vi "SP_ZAction.vi"(8 "error in (no error)":errorcluster, 10 "Z Action":T1(ring), 11 "SemiProbe in":refnum<class "SemiProbe.lvclass">) -> (0 "error out":errorcluster, 1 "previous Z [µm]":i32, 2 "Z [µm]":i32, 3 "SemiProbe out":refnum<class "SemiProbe.lvclass">)   [LabVIEW 2019, in "SemiProbe.lvclass"]
uses:
  SemiProbe.lvclass
  InstrumentSetup.vi
  <vilib>/Utility/error.llb/Error Cluster From Error Code.vi
  <vilib>/ErrorRing/Error Ring.xnode
  ArduinoControl/ArduinoControl.lvclass
  InstrControl.lvclass
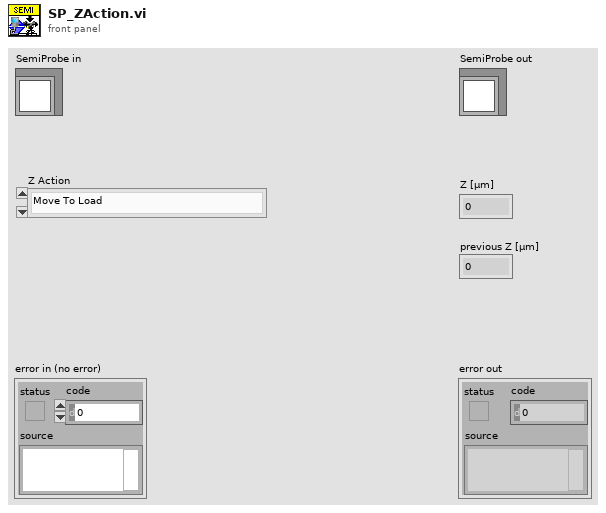
[diagram p1: front panel]
types:
  T1 = enum16{"Move To Load", "Move To Double Separation", "Move To Separation Distance", "Move To Contact", "Execute Contact Search", "Execute Arduino Contact Search"}
  T2 = cluster{"SP Load Less Than Thr?":bool, "SP Load Threshold (um)":dbl, "SP Current Location":cluster{"X (um)":ext, "Y (um)":ext, "Z (um)":ext, "T (degree)":ext}, "SP Chuck Speeds":cluster{"XY Speed (10-100%)":dbl, "Z Speed (10-100%)":dbl, "T Speed (10-100%)":dbl}, "Manual Step Parameters":cluster{"Step in X":bool, "X S-Speed [µm/step]":sgl, "Step in Y":bool, "Y S-Speed [µm/step]":sgl, "Step in Z":bool, "Z S-Speed [µm/step]":sgl, "Step in T":bool, "T S-Speed [mdegree/step]":sgl, "X Increase":bool, "Y Increase?":bool, "Z Increase?":bool, "T Increase?":bool}, "Z Stepper":cluster{"UP/DOWN":bool, "UP/DOWN Speed [µm/step]":i32, "SP Z Step":bool}, "Z Heights Set":bool, "SP Contact Search":cluster{"Contact Circuit":enum16{"12", "1", "2"}, "Speed [1000-10000]":sgl, "Start Height [µm]":sgl, "Search Band [µm]":sgl, "Overdrive [µm]":sgl}, "Separation Distance [µm]":u32, "Contact Height [µm]":u32, "Use Overdrive?":bool, "Touchdown method":enum16{"no feedback", "Arduino edgesense", "SP contact circuit"}, "Arduino Edgesense params":cluster{"touchdown height [µm]":i32, "search band [µm]":u32, "speed [µm/step]":u32, "overdrive [µm]":u32}}
  T3 = cluster{"Contact Circuit":enum16{"12", "1", "2"}, "Speed [1000-10000]":sgl, "Start Height [µm]":sgl, "Search Band [µm]":sgl, "Overdrive [µm]":sgl}
  T4 = cluster{"touchdown height [µm]":i32, "search band [µm]":u32, "speed [µm/step]":u32, "overdrive [µm]":u32}
  T5 = cluster{"VISA address":refnum<visa-resource-name>, "T sensor":enum16{"SHT", "DS"}, "Arduino":refnum<class "ArduinoControl.lvclass">}
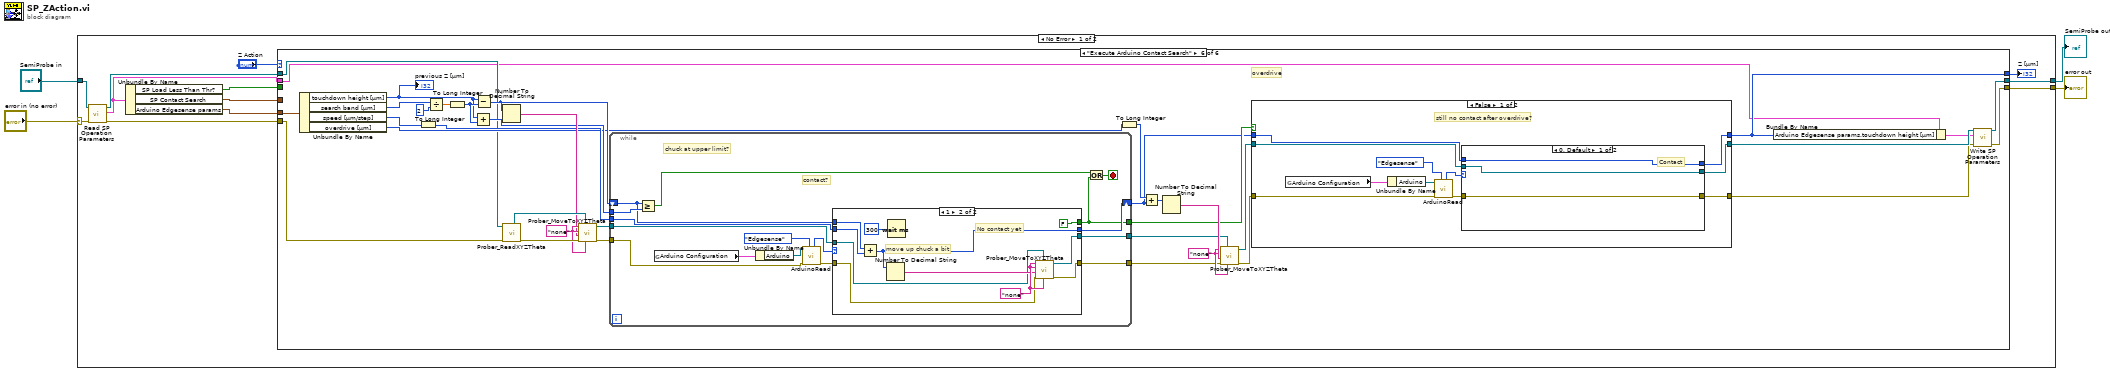
[diagram p0: block diagram]
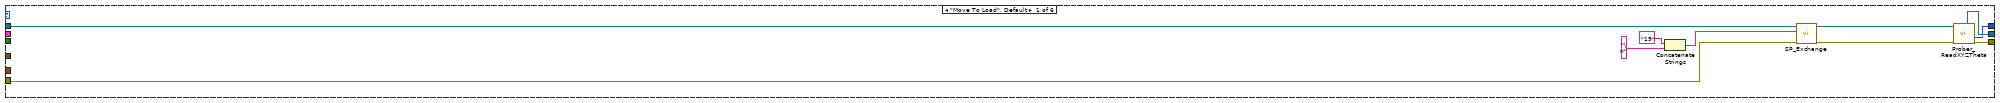
[diagram p2: hidden frame]
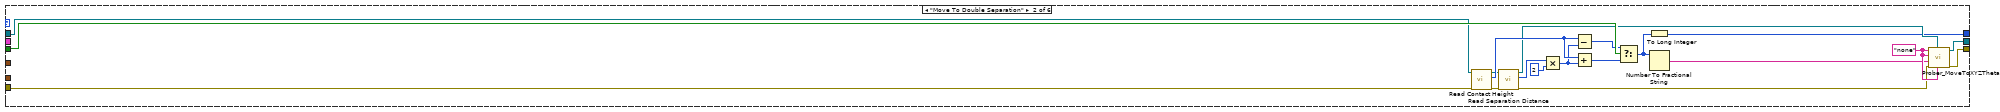
[diagram p3: hidden frame]
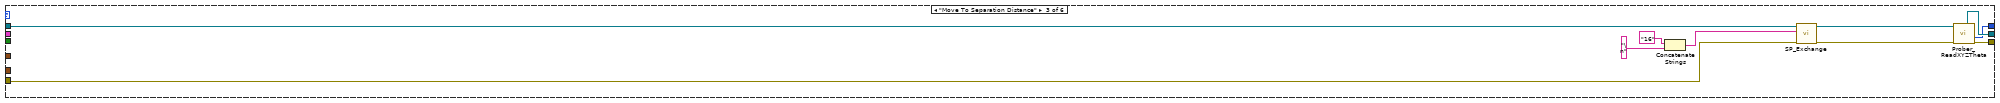
[diagram p4: hidden frame]
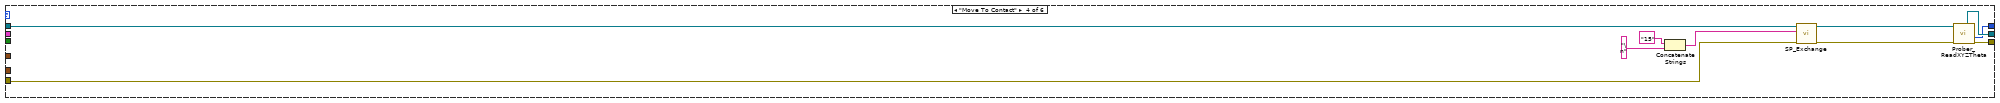
[diagram p5: hidden frame]
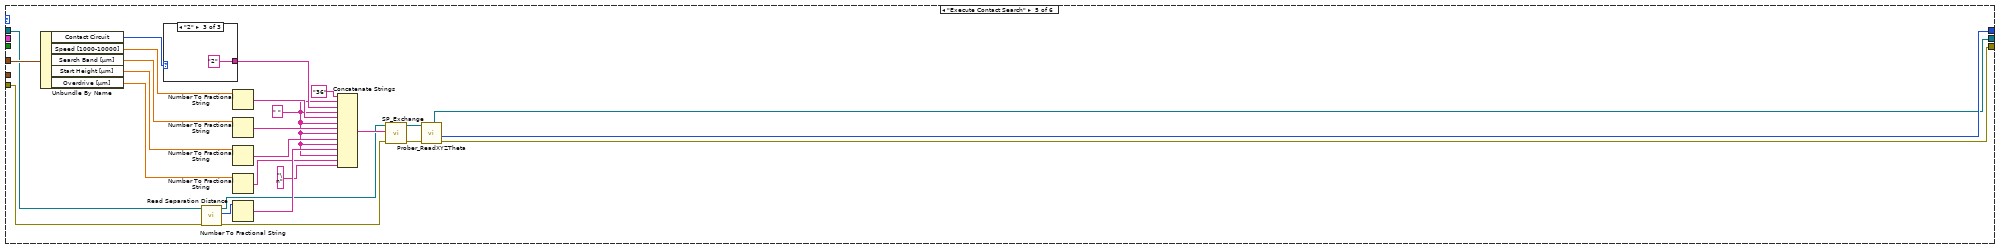
[diagram p6: hidden frame]
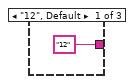
[diagram p7: hidden frame]
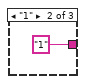
[diagram p8: hidden frame]
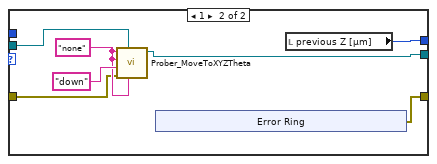
[diagram p9: hidden frame]
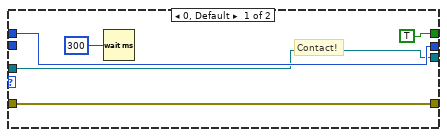
[diagram p11: hidden frame]
diagram:
  n1 = case shown="No Error" "error in (no error)" {
    selector: "error in (no error)" -> [w9 w193]
    tunnel: [w14 w193] -> w3
    tunnel: [w15 w192] -> w1
    tunnel: "SemiProbe in" -> [w13 w192]
    frame No Error {
      n2 = call-dynamic "Read SP Operation Parameters.vi"("error in (no error)"=w9, "SemiProbe in"=w13) -> ("error out"=w10:errorcluster, "SP Operation Parameters"=w5:T2, "SemiProbe out"=w11:refnum<class "SemiProbe.lvclass">)  [unwired: 7 in]
      n3 = Unbundle By Name(w5) -> ("SP Load Less Than Thr?"=w12:bool, "SP Contact Search"=w8:T3, "Arduino Edgesense params"=w6:T4)
      n4 = case shown="\"Execute Arduino Contact Search\"" "Z Action" {
        tunnel: [w20 w29 w50 w57 w69 w99] -> w15
        tunnel: [w21 w30 w47 w58 w71 w98] -> w14
        tunnel: w12 -> [_ w42 _ _ _ _]
        tunnel: w11 -> [w17 w35 w52 w62 w80 w103]
        tunnel: w10 -> [w18 w34 w51 w61 w79 w104]
        tunnel: w8 -> [_ _ _ _ w89 _]
        tunnel: [w19 w27 w46 w56 w70 w101] -> w7
        tunnel: w6 -> [_ _ _ _ _ w102]
        tunnel: w5 -> [_ _ _ _ _ w96]
        frame "Move To Load", Default {
          n5 = Concatenate Strings("19", "\n") -> (w24:string)
          n6 = call-dynamic "SP_Exchange.vi"("error in (no error)"=w18, "command"=w24, "SemiProbe in"=w17) -> ("error out"=w22:errorcluster, "SemiProbe out"=w23:refnum<class "SemiProbe.lvclass">)  [unwired: 4 in, 3 out]
          n7 = call-dynamic "Prober_ReadXYZTheta.vi"("error in (no error)"=w22, "SemiProbe in"=w23) -> ("error out"=w21:errorcluster, "Z location [µm]"=w19:i32, "SemiProbe out"=w20:refnum<class "SemiProbe.lvclass">)  [unwired: 4 in, 3 out]
        }
        frame "Move To Double Separation" {
          w45 = "none"
          n8 = call-dynamic "Read Contact Height.vi"("error in (no error)"=w34, "SemiProbe in"=w35) -> ("error out"=w36:errorcluster, "Contact Height [µm]"=w39:u32, "SemiProbe out"=w37:refnum<class "SemiProbe.lvclass">)  [unwired: 7 in]
          n9 = call-dynamic "Read Separation Distance.vi"("error in (no error)"=w36, "SemiProbe in"=w37) -> ("error out"=w33:errorcluster, "Separation Distance"=w43:u32, "SemiProbe out"=w31:refnum<class "SemiProbe.lvclass">)  [unwired: 7 in]
          n10 = Multiply(x=w43, y=2) -> (x*y=w38:u32)
          n11 = Subtract(x=w39, y=w38) -> (x-y=w41:u32)
          n12 = Add(x=w39, y=w38) -> (x+y=w40:u32)
          n13 = Select(t=w41, s=w42, f=w40) -> (s? t:f=w28:u32)
          n14 = To Long Integer(number=w28) -> (32bit integer=w27:i32)
          n15 = Number To Fractional String(number=w28) -> (F-format string=w32:string)  [unwired: 3 in]
          n16 = call-dynamic "Prober_MoveToXYZTheta.vi"("Theta location [mdeg]"=w45, "SemiProbe in"=w31, "error in (no error)"=w33, "Z location [µm]"=w32, "Y location [µm]"=w45, "X location [µm]"=w45) -> ("error out"=w30:errorcluster, "SemiProbe out"=w29:refnum<class "SemiProbe.lvclass">)  [unwired: 3 in, 1 out]
        }
        frame "Move To Separation Distance" {
          n17 = Concatenate Strings("16", "\n") -> (w53:string)
          n18 = call-dynamic "SP_Exchange.vi"("error in (no error)"=w51, "command"=w53, "SemiProbe in"=w52) -> ("error out"=w48:errorcluster, "SemiProbe out"=w49:refnum<class "SemiProbe.lvclass">)  [unwired: 4 in, 3 out]
          n19 = call-dynamic "Prober_ReadXYZTheta.vi"("error in (no error)"=w48, "SemiProbe in"=w49) -> ("error out"=w47:errorcluster, "Z location [µm]"=w46:i32, "SemiProbe out"=w50:refnum<class "SemiProbe.lvclass">)  [unwired: 4 in, 3 out]
        }
        frame "Move To Contact" {
          n20 = Concatenate Strings("15", "\n") -> (w63:string)
          n21 = call-dynamic "SP_Exchange.vi"("error in (no error)"=w61, "command"=w63, "SemiProbe in"=w62) -> ("error out"=w59:errorcluster, "SemiProbe out"=w60:refnum<class "SemiProbe.lvclass">)  [unwired: 4 in, 3 out]
          n22 = call-dynamic "Prober_ReadXYZTheta.vi"("error in (no error)"=w59, "SemiProbe in"=w60) -> ("error out"=w58:errorcluster, "Z location [µm]"=w56:i32, "SemiProbe out"=w57:refnum<class "SemiProbe.lvclass">)  [unwired: 4 in, 3 out]
        }
        frame "Execute Contact Search" {
          w74 = " "
          n23 = Unbundle By Name(w89) -> ("Contact Circuit"=w88:enum16{"12", "1", "2"}, "Speed [1000-10000]"=w86:sgl, "Search Band [µm]"=w85:sgl, "Start Height [µm]"=w84:sgl, "Overdrive [µm]"=w68:sgl)
          n24 = case shown="\"2\"" w88 {
            tunnel: ["12" "1" "2"] -> w87
            frame "12", Default {
            }
            frame "1" {
            }
            frame "2" {
            }
          }
          n25 = call-dynamic "Read Separation Distance.vi"("error in (no error)"=w79, "SemiProbe in"=w80) -> ("error out"=w67:errorcluster, "Separation Distance"=w78:u32, "SemiProbe out"=w66:refnum<class "SemiProbe.lvclass">)  [unwired: 7 in]
          n26 = Number To Fractional String(number=w86) -> (F-format string=w83:string)  [unwired: 3 in]
          n27 = Number To Fractional String(number=w85) -> (F-format string=w82:string)  [unwired: 3 in]
          n28 = Number To Fractional String(number=w84) -> (F-format string=w81:string)  [unwired: 3 in]
          n29 = Number To Fractional String(number=w68) -> (F-format string=w76:string)  [unwired: 3 in]
          n30 = Number To Fractional String(number=w78) -> (F-format string=w77:string)  [unwired: 3 in]
          n31 = Concatenate Strings("36", w74, w87, w74, w83, w74, w82, w74, w81, w74, w77, w74, w76, "\n") -> (w90:string)
          n32 = call-dynamic "SP_Exchange.vi"("error in (no error)"=w67, "command"=w90, "SemiProbe in"=w66) -> ("error out"=w72:errorcluster, "SemiProbe out"=w73:refnum<class "SemiProbe.lvclass">)  [unwired: 4 in, 3 out]
          n33 = call-dynamic "Prober_ReadXYZTheta.vi"("error in (no error)"=w72, "SemiProbe in"=w73) -> ("error out"=w71:errorcluster, "Z location [µm]"=w70:i32, "SemiProbe out"=w69:refnum<class "SemiProbe.lvclass">)  [unwired: 4 in, 3 out]
        }
        frame "Execute Arduino Contact Search" {
          w112 = "none" ("Z location")
          w123 = "none" ("Z location")
          # "overdrive"
          n34 = Unbundle By Name(w102) -> ("touchdown height [µm]"=w105:i32, "search band [µm]"=w129:u32, "speed [µm/step]"=w130:u32, "overdrive [µm]"=w116:u32)
          "previous Z [µm]" <- w105
          n35 = To Long Integer(number=w130) -> (32bit integer=w117:i32)
          n36 = Divide(x=w129, y=u32 2) -> (x/y=w127:dbl)
          n37 = To Long Integer(number=w127) -> (32bit integer=w126:i32)
          n38 = Add(x=w105, y=w126) -> (x+y=w121:i32)
          n39 = Subtract(x=w105, y=w126) -> (x-y=w120:i32)
          n40 = Number To Decimal String(number=w120) -> (decimal integer string=w122:string)  [unwired: 1 in]
          n41 = call-dynamic "Prober_ReadXYZTheta.vi"("error in (no error)"=w104, "SemiProbe in"=w103) -> ("error out"=w124:errorcluster, "SemiProbe out"=w125:refnum<class "SemiProbe.lvclass">)  [unwired: 4 in, 4 out]
          n42 = call-dynamic "Prober_MoveToXYZTheta.vi"("Theta location [mdeg]"=w123, "SemiProbe in"=w125, "error in (no error)"=w124, "Z location [µm]"=w122, "Y location [µm]"=w123, "X location [µm]"=w123) -> ("error out"=w119:errorcluster, "SemiProbe out"=w118:refnum<class "SemiProbe.lvclass">)  [unwired: 3 in, 1 out]
          n43 = while {
            tunnel: w121 -> [w170]
            shift-right: [w163] -> w106
            shift-left: w120 -> [w166]
            tunnel: w119 -> [w172]
            tunnel: w118 -> [w171]
            tunnel: w117 -> [w164]
            tunnel: [w162] -> w109
            tunnel: [w161] -> w111
            tunnel: [w160] -> w110
            stop <- w168 stop-if-true
            # "chuck at upper limit?"
            # "contact?"
            n44 = Greater Or Equal?(x=w166, y=w170) -> (x >= y?=w169:bool)
            n45 = global read "InstrumentSetup.vi" "Arduino Configuration"() -> (w175:T5)
            n46 = Unbundle By Name(w175) -> ("Arduino"=w174:refnum<class "ArduinoControl.lvclass">)
            n47 = call "ArduinoRead.vi"("Arduino function"=enum16{"T/RH", "Interlock", "Edgesense"}."Edgesense", "error in (no error)"=w172, "ArduinoControl in"=w174) -> ("error out"=w165:errorcluster, "Edgesense Status"=w167:u16)  [unwired: 3 in, 4 out]
            n48 = case shown="1" w167 {
              tunnel: w164 -> [_ w191]
              tunnel: w166 -> [w177 w182]
              tunnel: [w177 w181] -> w163
              tunnel: [TRUE FALSE] -> w162
              tunnel: w165 -> [w179 w187]
              tunnel: [w179 w186] -> w161
              tunnel: w171 -> [w176 w184]
              tunnel: [w176 w183] -> w160
              frame 0, Default {
                # "Contact!"
                n49 = Wait (ms)(milliseconds to wait=300) -> ()  [unwired: 1 out]
              }
              frame 1 {
                w189 = "none" ("Z location")
                # "No contact yet"
                # "move up chuck a bit"
                n50 = Add(x=w182, y=w191) -> (x+y=w181:i32)
                n51 = Number To Decimal String(number=w181) -> (decimal integer string=w188:string)  [unwired: 1 in]
                n52 = Wait (ms)(milliseconds to wait=300) -> ()  [unwired: 1 out]
                n53 = call-dynamic "Prober_MoveToXYZTheta.vi"("Theta location [mdeg]"=w189, "SemiProbe in"=w184, "error in (no error)"=w187, "Z location [µm]"=w188, "Y location [µm]"=w189, "X location [µm]"=w189) -> ("error out"=w186:errorcluster, "SemiProbe out"=w183:refnum<class "SemiProbe.lvclass">)  [unwired: 3 in, 1 out]
              }
            }
            n54 = Or(x=w169, y=w162) -> (x .or. y?=w168:bool)
          }
          n55 = To Long Integer(number=w116) -> (32bit integer=w115:i32)
          n56 = Add(x=w115, y=w106) -> (x+y=w114:i32)
          n57 = Number To Decimal String(number=w114) -> (decimal integer string=w113:string)  [unwired: 1 in]
          n58 = call-dynamic "Prober_MoveToXYZTheta.vi"("Theta location [mdeg]"=w112, "SemiProbe in"=w110, "error in (no error)"=w111, "Z location [µm]"=w113, "Y location [µm]"=w112, "X location [µm]"=w112) -> ("error out"=w107:errorcluster, "SemiProbe out"=w108:refnum<class "SemiProbe.lvclass">)  [unwired: 3 in, 1 out]
          n59 = case shown="False" w109 {
            tunnel: w108 -> [w135 w157]
            tunnel: w107 -> [w139 w158]
            tunnel: w106 -> [w134 w159]
            tunnel: [w133 w158] -> w97
            tunnel: [w132 w159] -> w101
            tunnel: [w131 w157] -> w100
            frame False {
              # "still no contact after overdrive?"
              n60 = global read "InstrumentSetup.vi" "Arduino Configuration"() -> (w141:T5)
              n61 = Unbundle By Name(w141) -> ("Arduino"=w140:refnum<class "ArduinoControl.lvclass">)
              n62 = call "ArduinoRead.vi"("Arduino function"=enum16{"T/RH", "Interlock", "Edgesense"}."Edgesense", "error in (no error)"=w139, "ArduinoControl in"=w140) -> ("error out"=w137:errorcluster, "Edgesense Status"=w136:u16)  [unwired: 3 in, 4 out]
              n63 = case shown="0, Default" w136 {
                tunnel: w137 -> [w143 w149]
                tunnel: w135 -> [w144 w148]
                tunnel: w134 -> [w142 _]
                tunnel: [w143 w147] -> w133
                tunnel: [w142 w146] -> w132
                tunnel: [w144 w145] -> w131
                frame 0, Default {
                  # "Contact"
                }
                frame 1 {
                  w150 = "none" ("Z location")
                  n64 = call-dynamic "Prober_MoveToXYZTheta.vi"("Theta location [mdeg]"=w150, "SemiProbe in"=w148, "error in (no error)"=w149, "Z location [µm]"="down", "Y location [µm]"=w150, "X location [µm]"=w150) -> ("SemiProbe out"=w145:refnum<class "SemiProbe.lvclass">)  [unwired: 3 in, 2 out]
                  n65 = xnode "Error Ring"() -> ("error out"=w147:errorcluster)
                  n66 = local read "previous Z [µm]"() -> (w146:i32)
                }
              }
            }
            frame True {
            }
          }
          n67 = Bundle By Name(cluster=w96, "Arduino Edgesense params.touchdown height [µm]"=w101) -> (w95:T2)
          n68 = call-dynamic "Write SP Operation Parameters.vi"("error in (no error)"=w97, "SP Operation Parameters"=w95, "SemiProbe in"=w100) -> ("error out"=w98:errorcluster, "SemiProbe out"=w99:refnum<class "SemiProbe.lvclass">)  [unwired: 7 in]
        }
      }
      "Z [µm]" <- w7
    }
    frame Error {
    }
  }
  "error out" <- w3
  "SemiProbe out" <- w1
